vi "read_eval_print.vi"(10 "Environment in":T1, 11 "input string":string="(do \n  (eval (load \"~/repos/labview_lisp/lib/standard-lib.lablisp\"))\n  \n  (number? \"test\")\n)") -> (2 "Environment out":T1, 3 "expression out":string)   [LabVIEW 2020]
uses:
  ExpressionType.ctl
  Expression.ctl
  Environment.ctl
panel:
  in  "ShowType?":bool=TRUE
  out "Expression in":T2
  out "Expression out":T2
  out "expression in":string
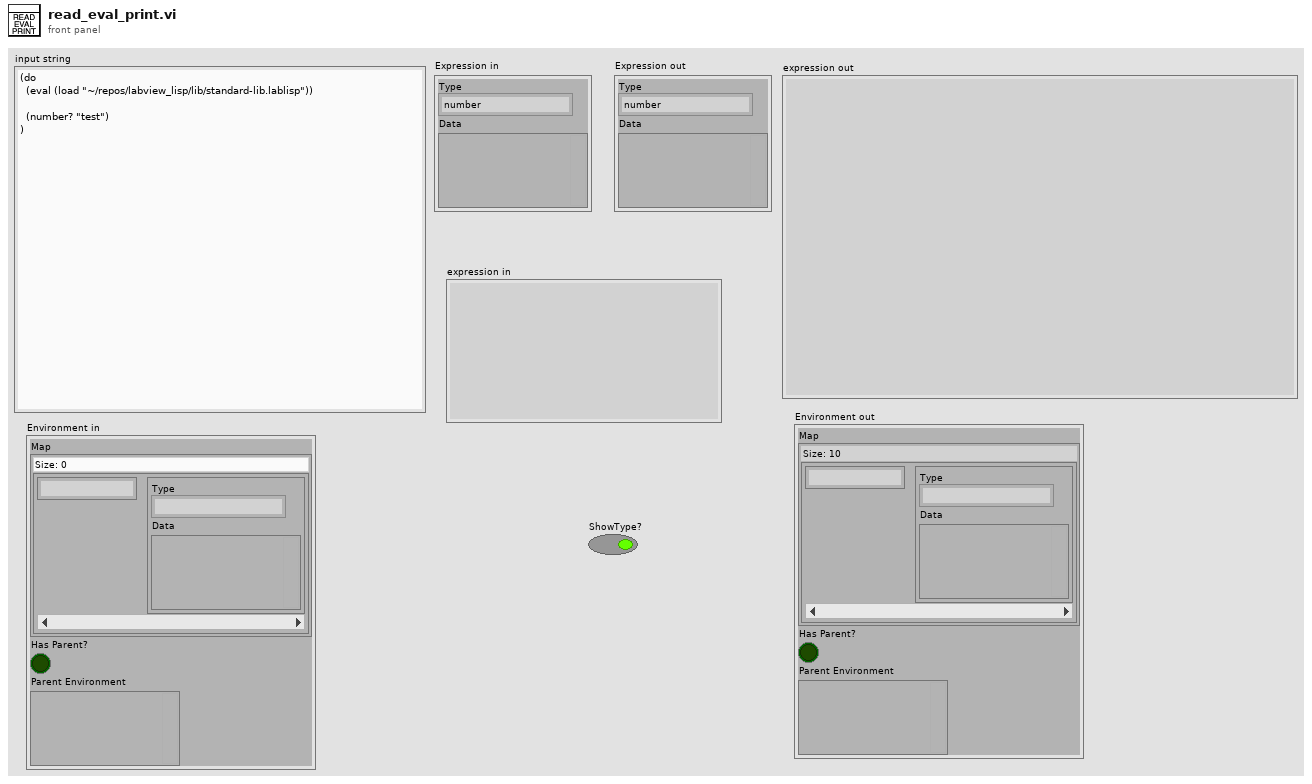
[diagram p1: front panel]
types:
  T1 = typedef "Environment.ctl" = cluster{"Map":map{string, T2}, "Has Parent?":bool, "Parent Environment":variant}
  T2 = typedef "Expression.ctl" = cluster{"Type":T3, "Data":variant}
  T3 = typedef "ExpressionType.ctl" = enum16{"number", "string", "symbol", "primitive", "list", "closure", "macro", "nil", "error"}
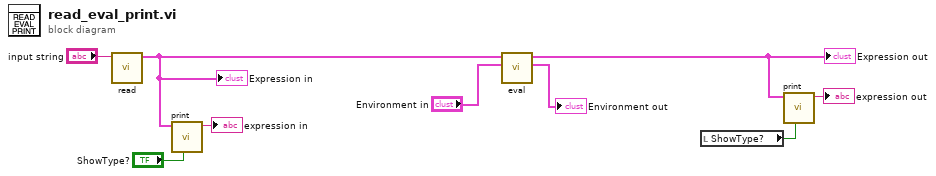
[diagram p0: block diagram]
diagram:
  n1 = call "read.vi"("input string"="input string") -> ("Expression out"=w7:T2)  [unwired: 10 in]
  "Expression in" <- w7
  n2 = call "print.vi"("ShowType?"="ShowType?", "Expression"=w7) -> ("String"=→"expression in":string)  [unwired: 8 in, 1 out]
  n3 = call "eval.vi"("Environment in"="Environment in", "Expression in"=w7) -> ("Environment out"=→"Environment out":T1, "Expression out"=w8:T2)  [unwired: 6 in]
  "Expression out" <- w8
  n4 = local read "ShowType?"() -> (w6:bool)
  n5 = call "print.vi"("ShowType?"=w6, "Expression"=w8) -> ("String"=→"expression out":string)  [unwired: 8 in, 1 out]
